vi "TCP_connect.vi"(8 "error in (no error)":errorcluster, 9 "IP address to listen on\n(blank to allow all networks)":string, 10 "port":u16=9000, 11 "TCP_IP.lvclass (in)":refnum<class "TCP_IP.lvclass">) -> (0 "error out":errorcluster)   [LabVIEW 2014, in "TCP_IP.lvclass"]
uses:
  TCP_IP.lvclass
  Globals.vi
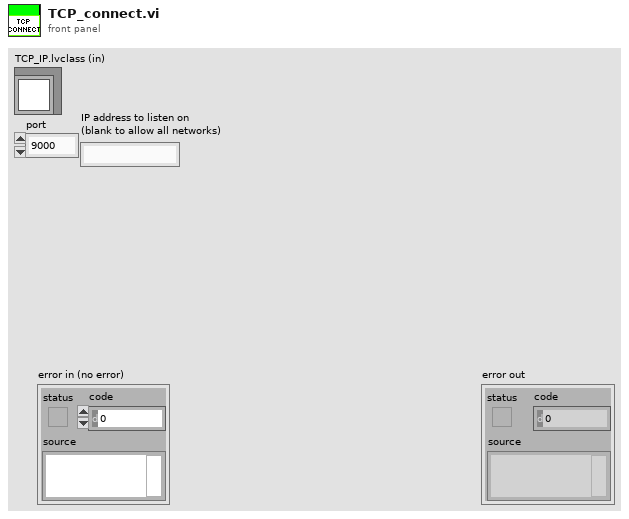
[diagram p1: front panel]
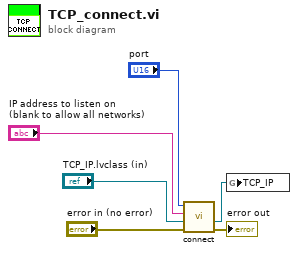
[diagram p0: block diagram]
diagram:
  n1 = call "connect.vi"("error in (no error)"="error in (no error)", "TCP_IP.lvclass (in)"="TCP_IP.lvclass (in)", "IP address to listen on\n(blank to allow all networks)"="IP address to listen on\n(blank to allow all networks)", "port"="port") -> ("error out"=→"error out":errorcluster, "TCP_IP.lvclass"=w2:refnum<class "TCP_IP.lvclass">)  [unwired: 6 in]
  n2 = global write "Globals.vi" "TCP_IP"(w2) -> ()
